vi "SVA 4MV6 P03 CCE RRMA .vi"() -> ()   [LabVIEW 2020]
doc: "Ceballos Conde Emanuel Rodríguez Ramírez Miguel Ángel 4MV6 Sistemas de visión artificial 2022/1\nEste vi permite reconocer objetos que se encuentren en la imagen obtenida siempre y cuando estos se encuentren guardados en la memoria de la neurona compet"
uses:
  <vilib>/userDefined/High Color/IMAQdx.ctl
  SVA 4MV6 P03 CCE RRMA.ctl
  <vilib>/vision/driver/IMAQdx.llb/IMAQdx Buffer Number Mode.ctl
  <vilib>/vision/driver/NI_Vision_Acquisition_Software.lvlib
panel:
  out "imagen binaria":T1(plugin-control)
  out "Deteccion de objeto":bool
  out "MOMENTOS INVARIANTES DE HU":dbl[](array[numeric])
  out "Objeto":string
  in  "UMBRAL":u8(knob)=150 scale=0.0..255.0
  in  "stop":bool
  out "video":T1(plugin-control)
  in  "Session In":T2
  # "Ceballos Conde Emanuel\nRodríguez Ramírez Miguel Ángel\n4MV6\nSistemas de visión artificial\n2022/1"
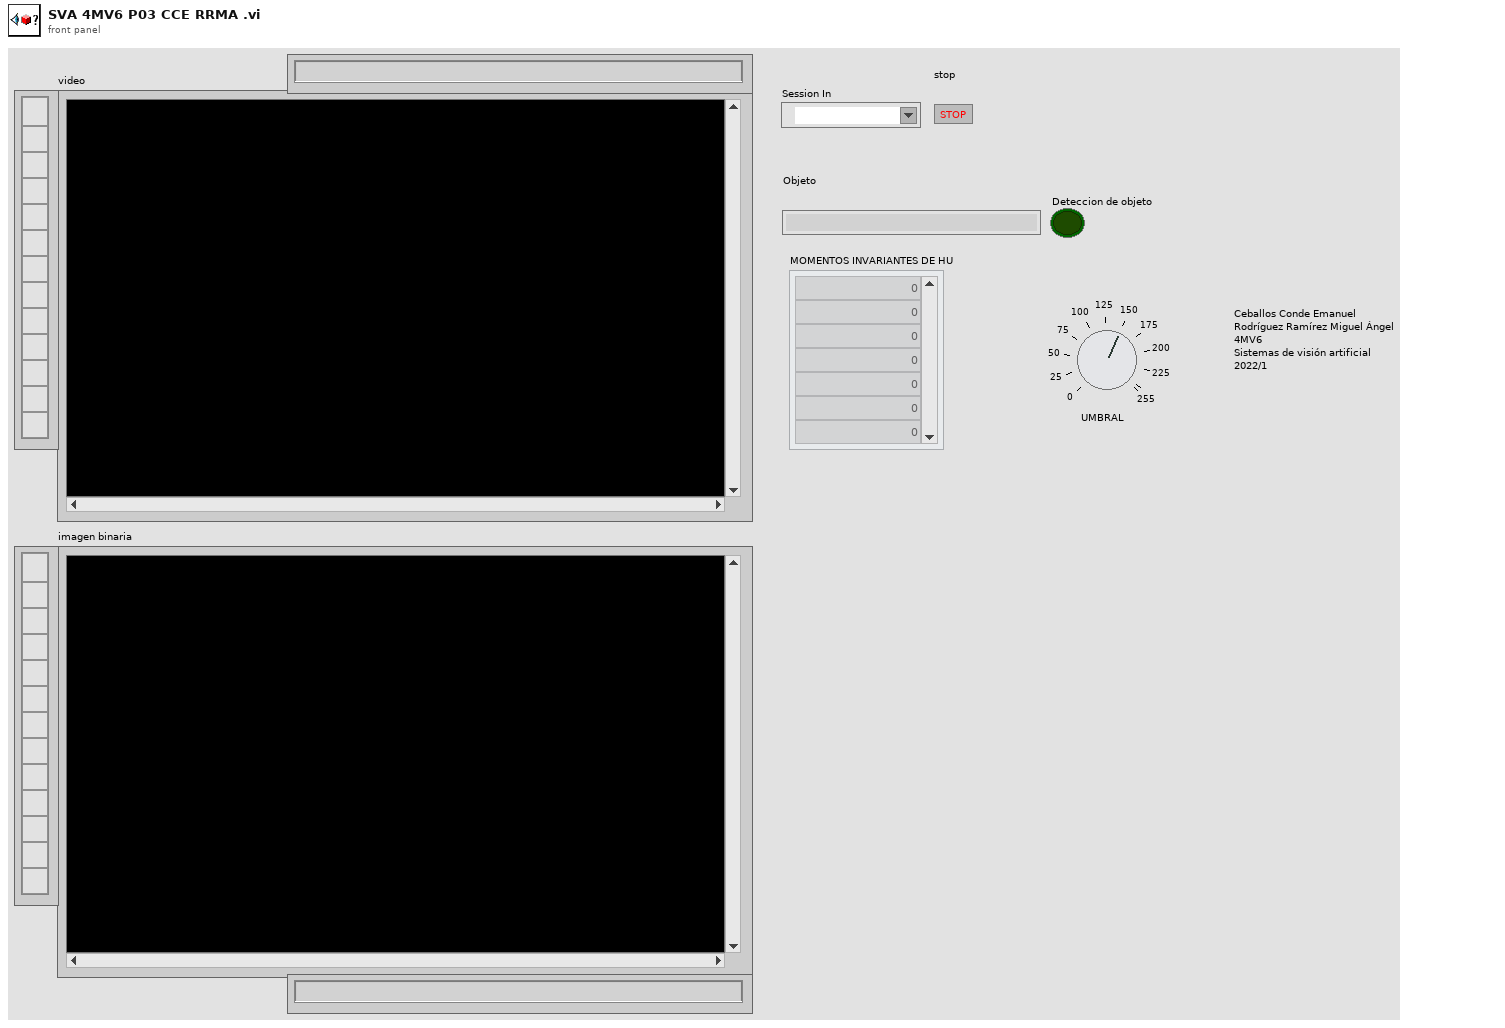
[diagram p1: front panel]
types:
  T1 = typedef "IMAQ Image.ctl" = refnum<image>
  T2 = typedef "IMAQdx.ctl" = refnum<k21>
  T3 = typedef "Image Type" = u32
  T4 = typedef "SVA 4MV6 P03 CCE RRMA.ctl" = enum16{"espera", "captura", "reconocimiento"}
  T5 = enum16{"H", "S", "V", "C", "M", "Y", "R", "G", "B", "RGB2GRAY MATLAB"}
  T6 = typedef "NI_Vision_Acquisition_Software.lvlib/IMAQdx Buffer Number Mode.ctl" = enum32{"Next", "Last", "Buffer Number", "Every", "Last New"}
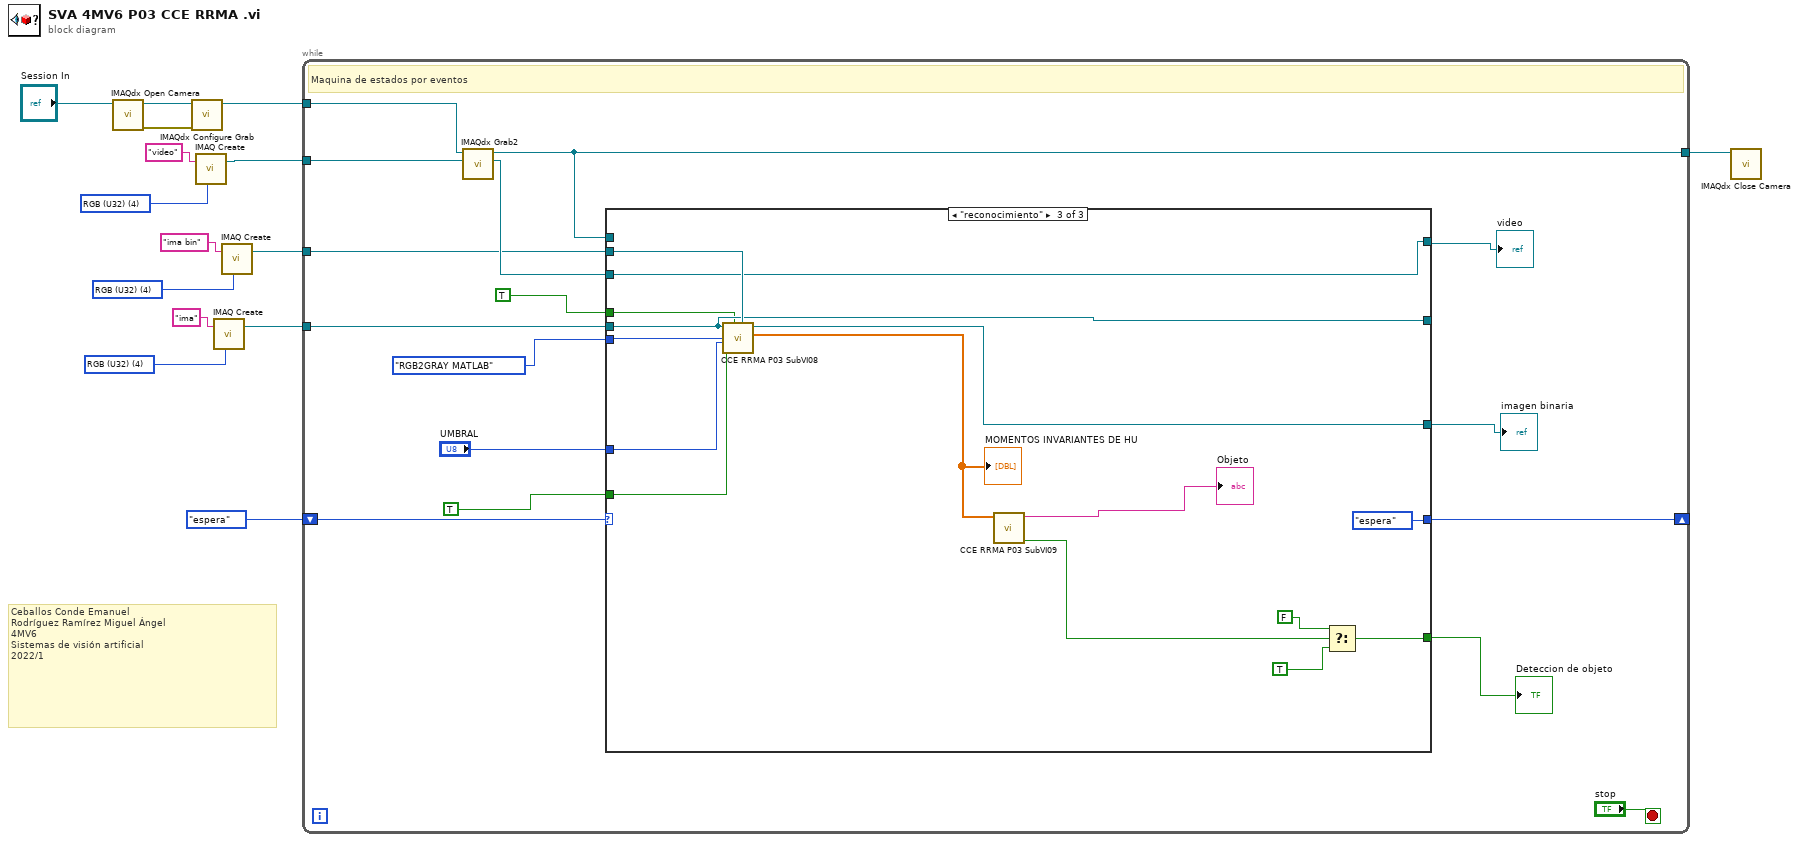
[diagram p0: block diagram]
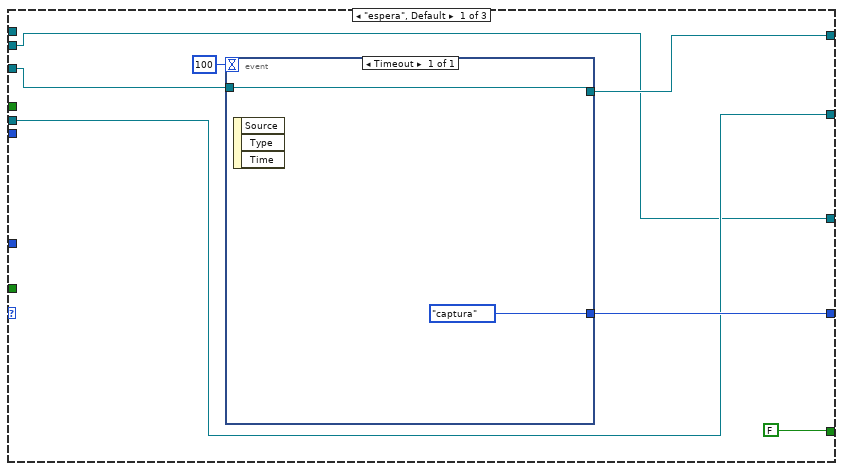
[diagram p2: hidden frame]
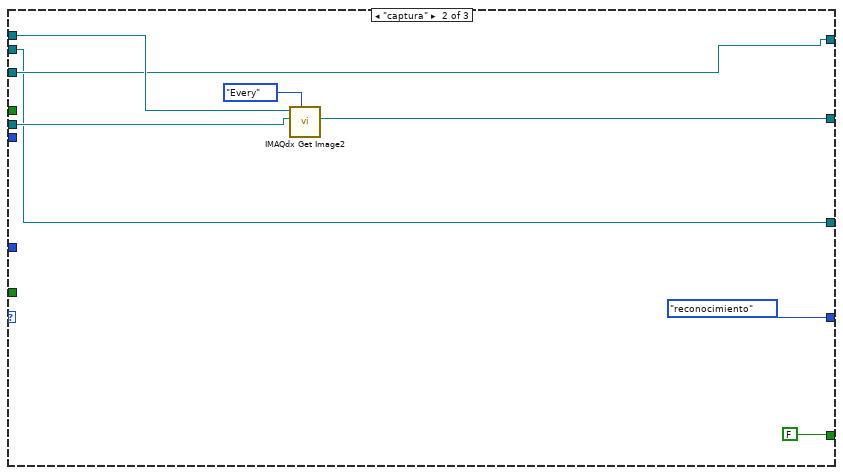
[diagram p3: hidden frame]
diagram:
  w2 = T3 4 items=["Grayscale (U8)", "Grayscale (I16)", "Grayscale (SGL)", "Complex (CSG)", "RGB (U32)", "HSL (U32)", "RGB (U64)", "Grayscale (U16)"] ("Image Type")
  w8 = T3 4 items=["Grayscale (U8)", "Grayscale (I16)", "Grayscale (SGL)", "Complex (CSG)", "RGB (U32)", "HSL (U32)", "RGB (U64)", "Grayscale (U16)"] ("Image Type")
  w10 = T3 4 items=["Grayscale (U8)", "Grayscale (I16)", "Grayscale (SGL)", "Complex (CSG)", "RGB (U32)", "HSL (U32)", "RGB (U64)", "Grayscale (U16)"] ("Image Type")
  # "Ceballos Conde Emanuel\nRodríguez Ramírez Miguel Ángel\n4MV6\nSistemas de visión artificial\n2022/1"
  n1 = call <vilib>:"IMAQdx Open Camera.vi"("Session In"="Session In") -> ("error out"=w13:errorcluster, "Session Out"=w14:T2)  [unwired: 9 in]
  n2 = call <vilib>:"IMAQdx Configure Grab.vi"("error in"=w13, "Session In"=w14) -> ("Session Out"=w7:T2)  [unwired: 8 in, 1 out]
  n3 = call "IMAQ Create"("Image Name"="video", "Image Type"=w10) -> ("New Image"=w6:T1)  [unwired: 3 in, 1 out]
  n4 = call "IMAQ Create"("Image Name"="ima", "Image Type"=w8) -> ("New Image"=w4:T1)  [unwired: 3 in, 1 out]
  n5 = call "IMAQ Create"("Image Name"="ima bin", "Image Type"=w2) -> ("New Image"=w1:T1)  [unwired: 3 in, 1 out]
  n6 = while {
    tunnel: w7 -> [w30]
    tunnel: w6 -> [w29]
    tunnel: [w28] -> w5
    tunnel: w4 -> [w27]
    shift-right: [w25] -> _
    shift-left: SVA_4MV6_P03_CCE_RRMA."espera" -> [w31]
    tunnel: w1 -> [w22]
    stop <- "stop" stop-if-true
    # "Maquina de estados por eventos"
    n7 = call <vilib>:"IMAQdx Grab2.vi"("Image In"=w29, "Session In"=w30) -> ("Image Out"=w26:T1, "Session Out"=w28:T2)  [unwired: 6 in, 2 out]
    n8 = case shown="\"reconocimiento\"" w31 {
      tunnel: w28 -> [_ w47 _]
      tunnel: w27 -> [w36 w46 w60]
      tunnel: w26 -> [w35 w45 w59]
      tunnel: [w34 w45 w59] -> w24
      tunnel: [w37 SVA_4MV6_P03_CCE_RRMA."reconocimiento" SVA_4MV6_P03_CCE_RRMA."espera"] -> w25
      tunnel: [w36 w44 w60] -> _
      tunnel: w22 -> [w33 w42 w62]
      tunnel: [w33 w42 w61] -> w16
      tunnel: T5."RGB2GRAY MATLAB" ("CAPA DE COLOR") -> [_ _ w58]
      tunnel: "UMBRAL" -> [_ _ w57]
      tunnel: TRUE ("INVERTIDO?") -> [_ _ w56]
      tunnel: TRUE ("NORMALIZACIÓN") -> [_ _ w55]
      tunnel: [FALSE FALSE w52] -> w17
      frame "espera", Default {
        n9 = event shown="[0] Timeout" {
          selector: _ -> [_]
          dyn-events: _ -> [_]
          timeout: 100 -> [_]
          tunnel: w35 -> [w39]
          tunnel: [SVA_4MV6_P03_CCE_RRMA."captura"] -> w37
          tunnel: [w39] -> w34
          event Timeout {
            n10 = event-data() -> ()  [unwired: 1 in, 3 out]
          }
        }
      }
      frame "captura" {
        n11 = call <vilib>:"IMAQdx Get Image2.vi"("Buffer Number Mode (Next)"=IMAQdx_Buffer_Number_Mode."Every", "Image In"=w46, "Session In"=w47) -> ("Image Out"=w44:T1)  [unwired: 5 in, 3 out]
      }
      frame "reconocimiento" {
        n12 = call "CCE RRMA P03 SubVI08.vi"("Image 3"=w62, "NORMALIZACIÓN"=w55, "INVERTIDO?"=w56, "UMBRAL"=w57, "CAPA DE COLOR"=w58, "Image"=w60) -> ("MOMENTOS INVARIANTES DE HU"=w51:dbl[], "Image 2"=w61:T1)  [unwired: 4 in]
        "MOMENTOS INVARIANTES DE HU" <- w51
        n13 = call "CCE RRMA P03 SubVI09.vi"("MOMENTOS INVARIANTES DE HU"=w51) -> ("logical OR"=w49:bool, "element"=→"Objeto":string)  [unwired: 7 in, 2 out]
        n14 = Select(t=FALSE, s=w49, f=TRUE) -> (s? t:f=w52:bool)
      }
    }
    "video" <- w24
    "Deteccion de objeto" <- w17
    "imagen binaria" <- w16
  }
  n15 = call <vilib>:"IMAQdx Close Camera.vi"("Session In"=w5) -> ()  [unwired: 10 in, 1 out]
